vi "CheckRedDAC.vi"(11 "amply":dbl) -> (2 "big":bool, 3 "ok":bool)   [LabVIEW 2012]
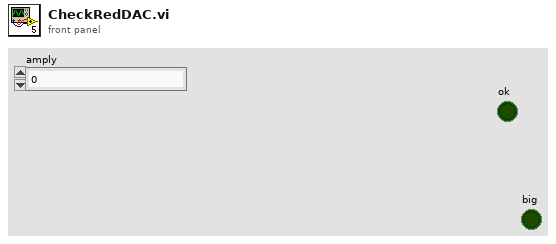
[diagram p1: front panel]
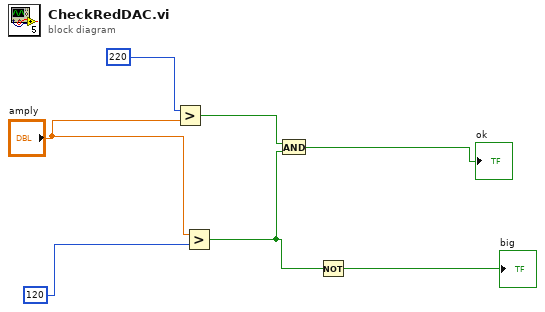
[diagram p0: block diagram]
diagram:
  n1 = Greater?(x=220, y="amply") -> (0:w4:bool)
  n2 = Greater?(x="amply", y=120) -> (0:w2:bool)
  n3 = And(x=w4, y=w2) -> (x .and. y?=→"ok":bool)
  n4 = Not(x=w2) -> (.not. x?=→"big":bool)
